vi "POST Multipart.vi"(6 "timeout (10000)":i32=10000, 7 "output file":path=path "", 8 "error in (no error)":errorcluster, 9 "data":T1[](array[typedef]), 10 "url":string, 11 "HTTP Client Abstract in":refnum<class "Abstract HTTP Client.lvclass">) -> (0 "error out":errorcluster, 1 "body":string, 2 "headers":string, 3 "HTTP Client Abstract out":refnum<class "Abstract HTTP Client.lvclass">)   [LabVIEW 2021, in "HTTP Client Abstract.lvlib" / "Abstract HTTP Client.lvclass"]
uses:
  Abstract HTTP Client.lvclass
  <vilib>/httpClient/MultipartData.ctl
  <vilib>/httpClient/LabVIEWHTTPClient.lvlib
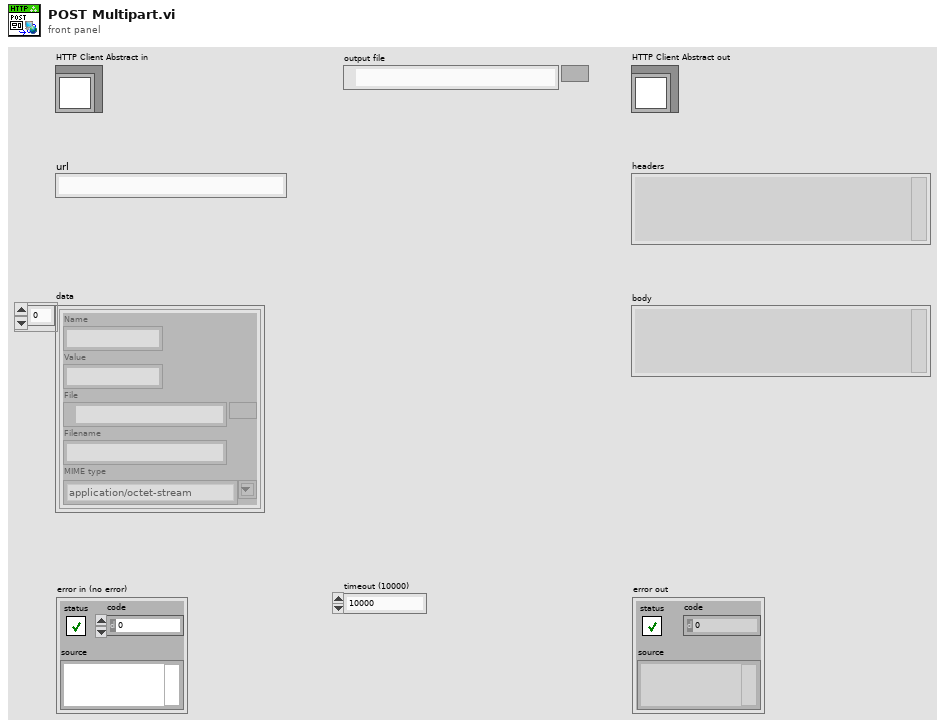
[diagram p1: front panel]
types:
  T1 = typedef "LabVIEWHTTPClient.lvlib/MultipartData.ctl" = cluster{"Name":string, "Value":string, "File":path, "Filename":string, "MIME type":string}
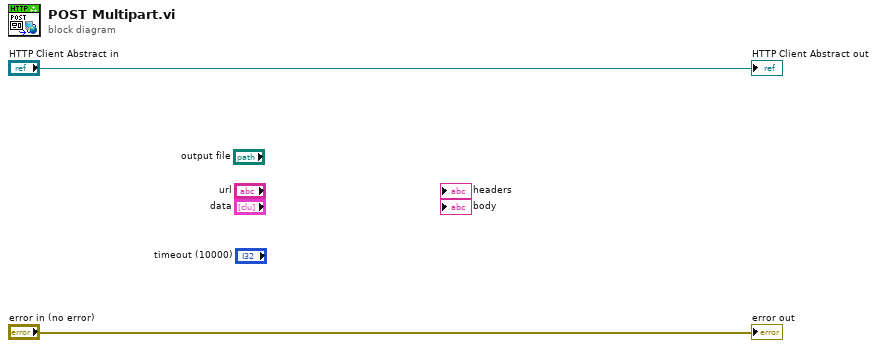
[diagram p0: block diagram]
diagram:
  "error out" <- "error in (no error)"
  "HTTP Client Abstract out" <- "HTTP Client Abstract in"
